vi "Configure Sequencer List All Increments.vi"(7 "List Increments":i32[](array[numeric]), 8 "error in (no error)":errorcluster, 10 "Instance (1)":i32=1, 11 "VISA resource name":refnum<visa-resource-name>) -> (0 "error out":errorcluster, 3 "VISA resource name out":refnum<visa-resource-name>)   [LabVIEW 2020, in "Rohde&Schwarz CMXP GPRF.lvlib"]
doc: "Defines the list increments for all sequencer list entries.\n\nAttribute:\nRSCMXPGPRF_ATTR_SEQUENCER_LIST_ALL_INCREMENTS\n\nRemote-control command:\nSOURce:GPRF:GEN<i>:SEQuencer:LIST:LINCrement:ALL"
uses:
  <instrlib>/Rohde&Schwarz CMXP GPRF/Rohde&Schwarz CMXP GPRF.lvlib
  <instrlib>/Rohde&Schwarz CMXP GPRF/Private/rsidr_core.llb/rsidr_core.lvlib
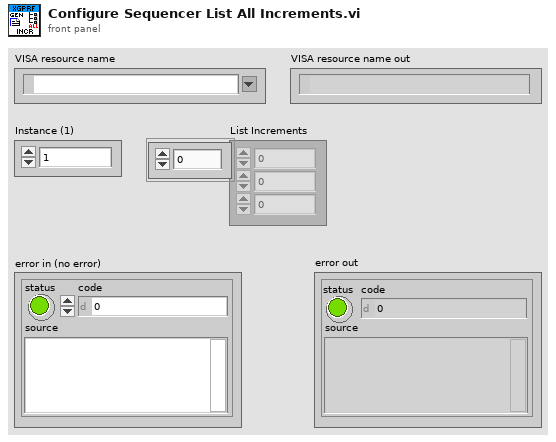
[diagram p1: front panel]
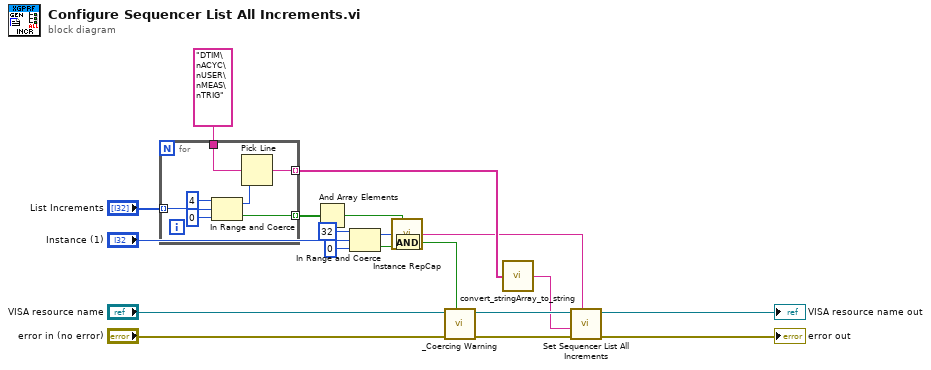
[diagram p0: block diagram]
diagram:
  n1 = for {
    tunnel: "List Increments" -> [w24] mode=indexing
    tunnel: "DTIM\nACYC\nUSER\nMEAS\nTRIG" ("format string") -> [w20]
    tunnel: [w26] -> w12 mode=indexing
    tunnel: [w22] -> w13 mode=indexing
    n2 = In Range and Coerce(upper limit=4, x=w24, lower limit=0) -> (coerced(x)=w21:i32, In Range?=w22:bool)
    n3 = Pick Line(multi-line string=w20, line index=w21) -> (output string=w26:string)  [unwired: 1 in]
  }
  n4 = And Array Elements(Boolean array=w13) -> (logical AND=w8:bool)
  n5 = In Range and Coerce(upper limit=32, x="Instance (1)", lower limit=0) -> (coerced(x)=w7:i32, In Range?=w9:bool)
  n6 = call <instrlib>:"Instance RepCap.vi"("Instance in"=w7) -> ("Instance out"=w2:string)
  n7 = And(x=w8, y=w9) -> (x .and. y?=w17:bool)
  n8 = call <instrlib>:"_Coercing Warning.vi"("In Range?"=w17, "error in (no error)"="error in (no error)", "VISA resource name"="VISA resource name") -> ("error out"=w6:errorcluster, "VISA resource name out"=w5:refnum<visa-resource-name>)  [unwired: 7 in]
  n9 = call <instrlib>:"convert_stringArray_to_string.vi"("string array in"=w12) -> ("string out"=w1:string)  [unwired: 4 in]
  n10 = call "Set Sequencer List All Increments"("Repeated Capabilities"=w2, "error in (no error)"=w6, "Sequencer List All Increments ()"=w1, "instrument handle"=w5) -> ("error out"=→"error out":errorcluster, "instrument handle out"=→"VISA resource name out":refnum<visa-resource-name>)  [unwired: 6 in]
